vi "niFpga wdp fft 4wire fifo.vi"(8 "read?":bool, 9 "write?":bool, 10 "data in im":fxp<+/-,8,1>[](array[numeric])=[0.0, 0.0], 11 "data in re":fxp<+/-,8,1>[](array[numeric])=[0.0, 0.0]) -> (2 "data out im":fxp<+/-,8,1>[](array[numeric]), 3 "data out re":fxp<+/-,8,1>[](array[numeric]))   [LabVIEW 2017]
uses:
  <vilib>/rvi/Emulation/niFpgaSctlEmulationGetInTimedLoop.vi
  <vilib>/Utility/error.llb/Clear Errors.vi
  <vilib>/rvi/DataTransferAndStorage/Container/Common/niFpgaContainerGetUniqueNameForEmu.vi
  <vilib>/rvi/DataTransferAndStorage/Container/Common/niFpgaContainerSetEmuInfo.vi
  <vilib>/rvi/eio/common/nirviEmuReportErrorAndStop.vi
  <vilib>/rvi/DataTransferAndStorage/Container/Common/niFpgaContainerExecOnDevCompGetState.vi
  <vilib>/rvi/Emulation/niFpgaEmulationIsFPGAContextNoSignature.vi
  <vilib>/rvi/errors/niFpgaSetErrorForExecOnDevCompSimple.vi
  <vilib>/rvi/FIFO/Fifo_Resource/nirvififoEmulationSetSize.vi
  <vilib>/rvi/FIFO/Fifo_Resource/nirviFifoEmulationQueueMgr.vi
  <instcachedir>/0/nirviFifoEmulationQueueMgr_E5CAEC123FF24DC58D834DCA3CDAA9B5.lvgen/nirviFifoEmulationQueueMgr_E5CAEC123FF24DC58D834DCA3CDAA9B5_001.vi
  <vilib>/rvi/FIFO/Fifo_Resource/nirvififoEmulationDetermineInputValidOut.vi
  <vilib>/rvi/FIFO/Fifo_Resource/nirvififoEmulationCreateLock.vi
  <vilib>/rvi/Emulation/niFpgaProcessEmulError.vi
  <vilib>/rvi/FIFO/Fifo_Resource/nirvififoEmulationObtainLock.vi
  <vilib>/rvi/FIFO/Fifo_Resource/nirvififoEmulationReleaseLock.vi
  <vilib>/rvi/occurrence/nirviWaitOnOccurrenceBase.vi
  <vilib>/rvi/errors/nirviReportUnexpectedCaseInternalError.vi
  <vilib>/rvi/errors/nirviReportUnexpectedCaseInternalError (U32).vi
  <vilib>/rvi/interface/RandomDataEmulation/niFpgaRandomDataHandleErrors.vi
  <vilib>/rvi/LocalResourceManager/LocalResourceManager.xnode
  <vilib>/rvi/DataTransferAndStorage/Container/XNode/niFpgaContainer.xnode
  <vilib>/rvi/FIFO/Fifo_Resource/niFpgaFifoEmulationRefIn.vi
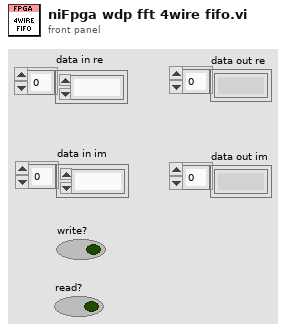
[diagram p1: front panel]
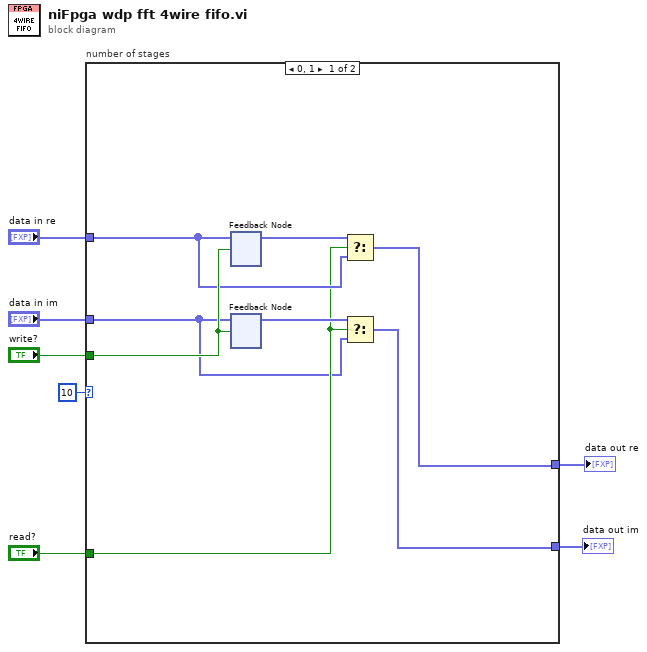
[diagram p0: block diagram]
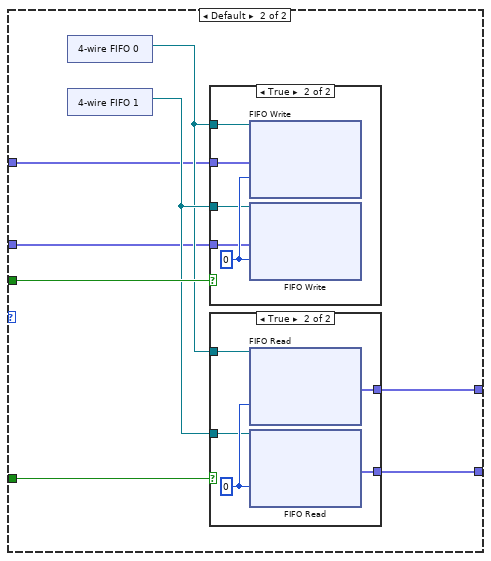
[diagram p2: hidden frame]
diagram:
  n1 = case "number of stages" shown="0, 1" u8 10 ("data in 0") {
    tunnel: [w9 w17] -> w2
    tunnel: "read?" -> [w11 w23]
    tunnel: "write?" -> [w15 w22]
    tunnel: "data in re" -> [w13 w19]
    tunnel: "data in im" -> [w10 w18]
    tunnel: [w8 w16] -> w1
    frame 0, 1 {
      n2 = feedback-in #1(w13, w15) -> ()
      n3 = feedback #1() -> (w14:fxp<+/-,8,1>[])  [unwired: 1 in]
      n4 = feedback #2() -> (w12:fxp<+/-,8,1>[])  [unwired: 1 in]
      n5 = feedback-in #2(w10, w15) -> ()
      n6 = Select(t=w14, s=w11, f=w13) -> (s? t:f=w9:fxp<+/-,8,1>[])
      n7 = Select(t=w12, s=w11, f=w10) -> (s? t:f=w8:fxp<+/-,8,1>[])
    }
    frame Default {
      n8 = xnode "4-wire FIFO 0"() -> ("FIFO Out"=w20:refnum<k21>)
      n9 = xnode "4-wire FIFO 1"() -> ("FIFO Out"=w21:refnum<k21>)
      n10 = case shown="True" w22 {
        tunnel: w19 -> [_ w32]
        tunnel: w18 -> [_ w31]
        tunnel: w20 -> [_ w30]
        tunnel: w21 -> [_ w29]
        frame False {
        }
        frame True {
          w33 = 0 ("Timeout")
          n11 = xnode ("FIFO Write")("Element"=w32, "Timeout"=w33, "FIFO In"=w30) -> ()  [unwired: 2 out]
          n12 = xnode ("FIFO Write")("Element"=w31, "Timeout"=w33, "FIFO In"=w29) -> ()  [unwired: 2 out]
        }
      }
      n13 = case shown="True" w23 {
        tunnel: [_ w27] -> w17
        tunnel: [_ w26] -> w16
        tunnel: w21 -> [_ w25]
        tunnel: w20 -> [_ w24]
        frame False {
        }
        frame True {
          w28 = 0 ("Timeout")
          n14 = xnode ("FIFO Read")("Timeout"=w28, "FIFO In"=w24) -> ("Element"=w27:fxp<+/-,8,1>[])  [unwired: 2 out]
          n15 = xnode ("FIFO Read")("Timeout"=w28, "FIFO In"=w25) -> ("Element"=w26:fxp<+/-,8,1>[])  [unwired: 2 out]
        }
      }
    }
  }
  "data out re" <- w2
  "data out im" <- w1
